vi "Robot Global Data.vi"() -> ()   [LabVIEW 2023]
doc: "This global VI can contain as many global variables as you need. To create a global variable, place a control on the panel, give it a good name. To read or write to it from a VI, drag the icon to the diagram of that VI. You can also drag from the project. Click on the node to change which global you access. You shouldn't have multiple locations writing to a global or it will cause a race-condition."
uses:
  <vilib>/Rock Robotics/WPI/Camera/WPI_CameraImageSize.ctl
  <vilib>/Rock Robotics/WPI/DriverStation/WPI_DriverStationRobotMode2.ctl
  Auto_Values.ctl
panel:
  out "Lift Lock":bool
  in  "Lift Right":dbl
  in  "Lift Left":dbl
  in  "Theta":dbl
  in  "Left Y":dbl
  in  "Left X":dbl
  in  "Robot Location":T1={"X Pos"=0.0, "Y Pos"=0.0, "Heading (Deg)"=0.0, "Strafe Throttle"=0.0, "Rot Throtle (Rad/s)"=0.0, "Strafe Tol (Ft)"=0.0, "Rotation Tol (Deg)"=0.0, "Shooter Pos"=enum."Travel", "Intake"=enum."Front", "Shooter Type"=enum."Manual", "Shooter Throttle"=0.0, "Wait (s)"=0.0, "Lift"=enum."Off"} {"Wait (s)" min=-360.0 max=360.0; "Rotation Tol (Deg)" min=-360.0 max=360.0; "Strafe Throttle" min=0.0 max=1.0}
  in  "Robot Setpoints":T1={"X Pos"=0.0, "Y Pos"=0.0, "Heading (Deg)"=0.0, "Strafe Throttle"=0.0, "Rot Throtle (Rad/s)"=0.0, "Strafe Tol (Ft)"=0.0, "Rotation Tol (Deg)"=0.0, "Shooter Pos"=enum."Travel", "Intake"=enum."Front", "Shooter Type"=enum."Manual", "Shooter Throttle"=0.0, "Wait (s)"=0.0, "Lift"=enum."Off"} {"Wait (s)" min=-360.0 max=360.0; "Rotation Tol (Deg)" min=-360.0 max=360.0; "Strafe Throttle" min=0.0 max=1.0}
  out "Auto Override":bool
  in  "Robot Mode":T2
  in  "image size":T3=enum."320x240"
  in  "Enable Vision":bool
  # "Takes precedence\nfrom Tol"
  # "Takes precedence\nfrom Tol"
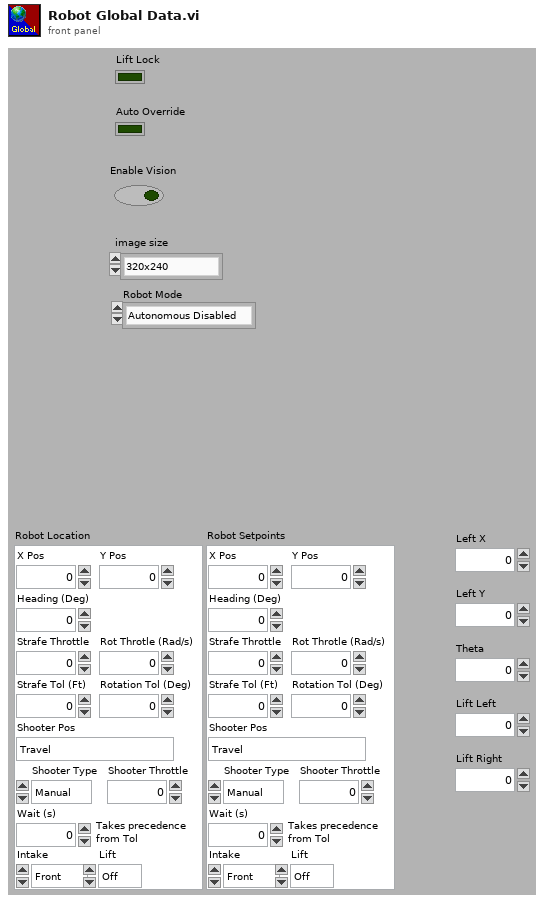
[diagram p1: front panel]
types:
  T1 = typedef "Auto_Values.ctl" = cluster{"X Pos":dbl, "Y Pos":dbl, "Heading (Deg)":dbl, "Strafe Throttle":dbl, "Rot Throtle (Rad/s)":dbl, "Strafe Tol (Ft)":dbl, "Rotation Tol (Deg)":dbl, "Shooter Pos":enum16{"Travel", "Speaker", "Amp"}, "Intake":enum16{"Off", "Front", "Center", "Out"}, "Shooter Type":enum16{"Off", "Manual", "Automatic"}, "Shooter Throttle":dbl, "Wait (s)":dbl, "Lift":enum16{"Off", "Up", "Down"}}
  T2 = typedef "WPI_DriverStationRobotMode2.ctl" = enum16{"Autonomous Disabled", "Autonomous Enabled", "Teleop Disabled", "Teleop Enabled", "Disconnected", "Finish", "Test Disabled", "Test Enabled", "Emergency Stopped"}
  T3 = typedef "WPI_CameraImageSize.ctl" = enum16{"640x480", "320x240", "160x120", "Custom"}
diagram:
